vi "Load Project from Path.vi"(8 "error in (no error)":errorcluster, 10 "Project Path":path, 11 "Model in":refnum<class "Model.lvclass">) -> (0 "error out":errorcluster, 3 "Model out":refnum<class "Model.lvclass">)   [LabVIEW 2015, in "Model.lvlib" / "Model.lvclass"]
uses:
  Model.lvclass
  Model Messages/Load Project from Reference Msg/Load Project from Reference Msg.lvclass
  <vilib>/ActorFramework/Actor/Actor.lvclass
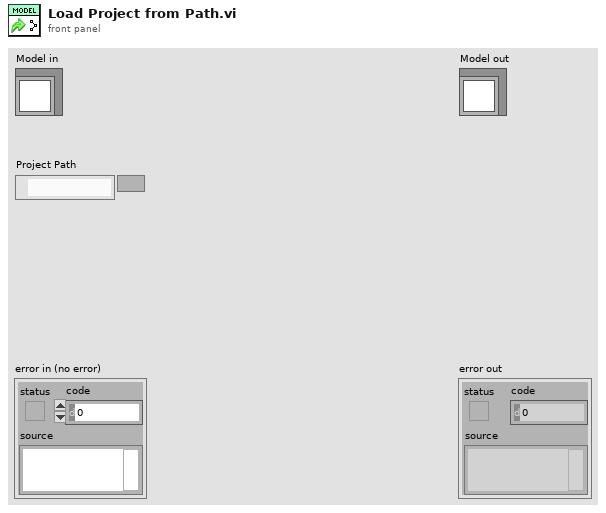
[diagram p1: front panel]
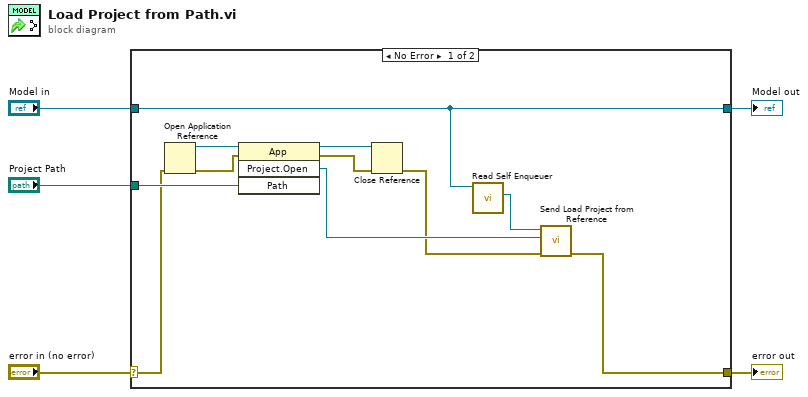
[diagram p0: block diagram]
diagram:
  n1 = case shown="No Error" "error in (no error)" {
    selector: "error in (no error)" -> [w13 w18]
    tunnel: [w8 w18] -> w4
    tunnel: [w7 w17] -> w2
    tunnel: "Model in" -> [w7 w17]
    tunnel: "Project Path" -> [w15 _]
    frame No Error {
      n2 = Open Application Reference(8:w13) -> (0:w14:errorcluster, 3:w16:refnum<vi>)  [unwired: 3 in]
      n3 = invoke class="App" method="Project.Open"(reference=w16, error in=w14, "Path"=w15) -> (reference out=w12:refnum<vi>, error out=w11:errorcluster, "Project:Open"=w10:refnum<vi>)  [unwired: 1 in, 1 out]
      n4 = Close Reference(reference=w12, error in (no error)=w11) -> (error out=w9:errorcluster)
      n5 = call <vilib>:"Read Self Enqueuer.vi"("Actor"=w7) -> ("Self Enqueuer"=w6:refnum<class "Message Enqueuer.lvclass">)  [unwired: 10 in]
      n6 = call "Send Load Project from Reference.vi"("error in (no error)"=w9, "Project Reference"=w10, "Message Enqueuer"=w6) -> ("error out"=w8:errorcluster)  [unwired: 7 in, 1 out]
    }
    frame Error {
    }
  }
  "error out" <- w4
  "Model out" <- w2
